vi "Labspec ConvertUnit.vi"(8 "error in":errorcluster, 9 "Direction":T1(ring), 10 "Initial Value":dbl, 11 "Automation Refnum In":refnum<k7>) -> (0 "error out":errorcluster, 2 "Converted Value":dbl, 3 "Automation Refnum Out":refnum<k7>)   [LabVIEW 2014]
panel:
  # "LICENSED MATERIALS – PROPERTY OF IBM\nCopyright IBM Corp. 2016,\nALL RIGHTS RESERVED"
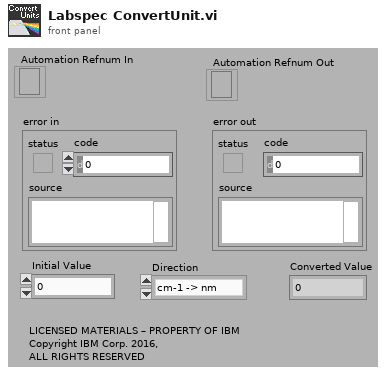
[diagram p1: front panel]
types:
  T1 = enum16{"cm-1 -> nm", "nm -> cm-1", "eV -> nm", "nm -> eV"}
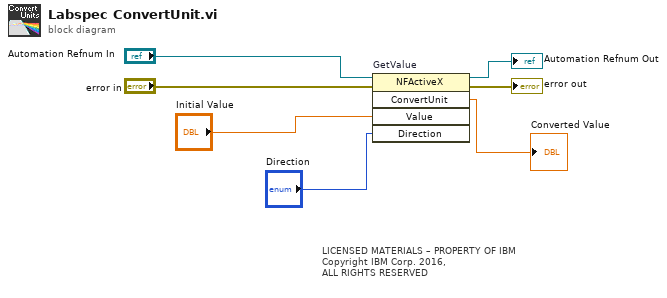
[diagram p0: block diagram]
diagram:
  # "LICENSED MATERIALS – PROPERTY OF IBM\nCopyright IBM Corp. 2016,\nALL RIGHTS RESERVED"
  n1 = invoke on="GetValue" class="NFActiveX" method="ConvertUnit"(reference="Automation Refnum In", error in="error in", "Value"="Initial Value", "Direction"="Direction") -> (reference out=→"Automation Refnum Out":refnum<k7>, error out=→"error out":errorcluster, "ConvertUnit"=→"Converted Value":dbl)  [unwired: 1 in, 2 out]
